vi "Sub01_CommandBuilder.vi"(8 "error in (no error)":errorcluster, 9 "CommandInfo":T1={"RedBall"={"Min"={"G"=0, "B"=0, "R"=160}, "Max"={"G"=160, "B"=160, "R"=255}}, "YellowBall"={"Min"={"G"=140, "B"=0, "R"=140}, "Max"={"G"=255, "B"=175, "R"=255}}, "WhiteBall"={"Min"={"G"=100, "B"=100, "R"=100}, "Max"={"G"=255, "B"=255, "R"=255}}, "BallDiameter"=11, "BackGround"={"Min"={"G"=91, "B"=202, "R"=39}, "Max"={"G"=116, "B"=255, "R"=62}}, "Border"={"Min"={"G"=0, "B"=121, "R"=0}, "Max"={"G"=42, "B"=126, "R"=14}}}, 10 "filenames":string[](array[string]), 11 "path in":path) -> (0 "error out":errorcluster, 3 "String":string)   [LabVIEW 2019]
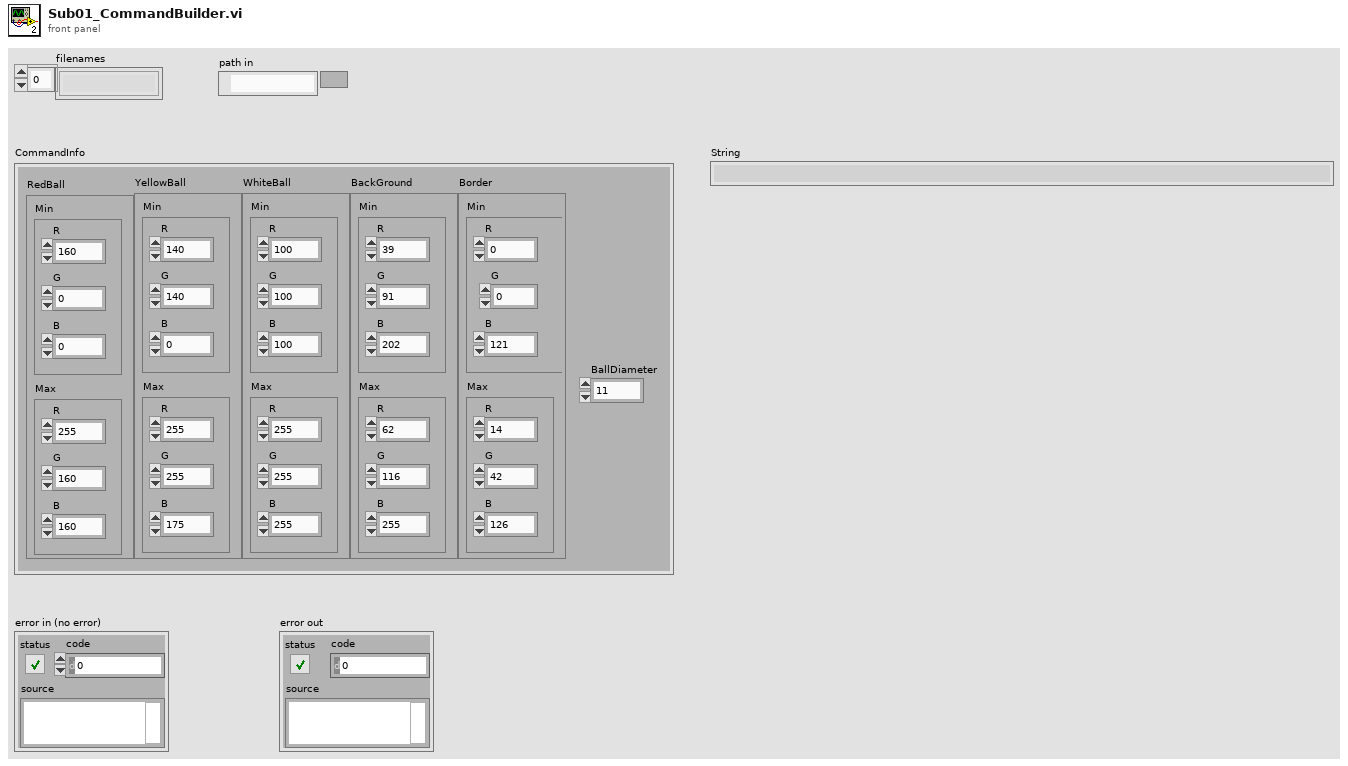
[diagram p1: front panel]
types:
  T1 = cluster{"RedBall":cluster{"Min":cluster{"G":u32, "B":u32, "R":u32}, "Max":cluster{"G":u32, "B":u32, "R":u32}}, "YellowBall":cluster{"Min":cluster{"G":u32, "B":u32, "R":u32}, "Max":cluster{"G":u32, "B":u32, "R":u32}}, "WhiteBall":cluster{"Min":cluster{"G":u32, "B":u32, "R":u32}, "Max":cluster{"G":u32, "B":u32, "R":u32}}, "BallDiameter":u32, "BackGround":cluster{"Min":cluster{"G":u32, "B":u32, "R":u32}, "Max":cluster{"G":u32, "B":u32, "R":u32}}, "Border":cluster{"Min":cluster{"G":u32, "B":u32, "R":u32}, "Max":cluster{"G":u32, "B":u32, "R":u32}}}
  T2 = cluster{"Min":cluster{"G":u32, "B":u32, "R":u32}, "Max":cluster{"G":u32, "B":u32, "R":u32}}
  T3 = typedef "imagedata.ctl" = cluster{"image type":i32, "image depth":i32, "image":u8[], "mask":u8[], "colors":u32[], "Rectangle":cluster{"left":i16, "top":i16, "right":i16, "bottom":i16}}
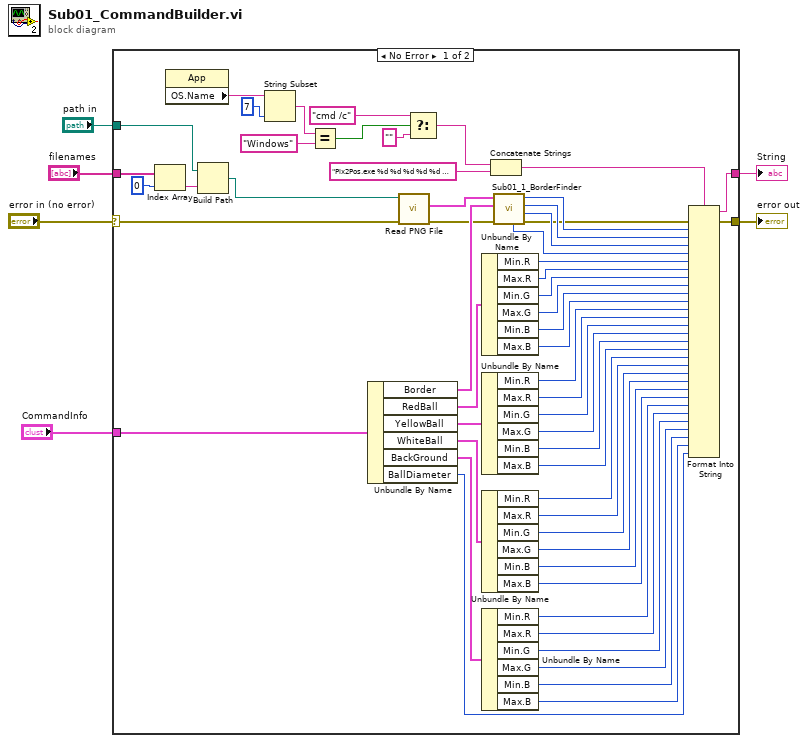
[diagram p0: block diagram]
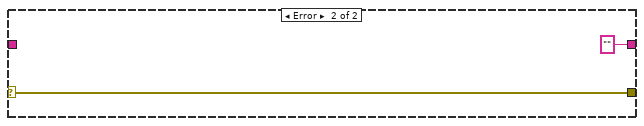
[diagram p2: hidden frame]
diagram:
  n1 = case shown="No Error" "error in (no error)" {
    selector: "error in (no error)" -> [w17 w63]
    tunnel: [w62 w63] -> w6
    tunnel: "filenames" -> [w59 _]
    tunnel: [w58 ""] -> w4
    tunnel: "CommandInfo" -> [w57 _]
    tunnel: "path in" -> [w18 _]
    frame No Error {
      n2 = Index Array(array=w59, index=0) -> (element=w54:string)
      n3 = property class="App"() -> ("OS.Name"=w9:string)  [unwired: 2 in, 2 out]
      n4 = Build Path(base path=w18, name or relative path=w54) -> (appended path=w61:path)
      n5 = String Subset(string=w9, length (rest)=7 ("length (rest)")) -> (substring=w7:string)  [unwired: 1 in]
      n6 = Equal?(x=w7, y="Windows") -> (x = y?=w12:bool)
      n7 = Unbundle By Name(w57) -> ("Border"=w56:T2, "RedBall"=w27:T2, "YellowBall"=w34:T2, "WhiteBall"=w35:T2, "BackGround"=w48:T2, "BallDiameter"=w55:u32)
      n8 = call <vilib>:"Read PNG File.vi"("error in (no error)"=w17, "path to PNG file"=w61) -> ("error out"=w20:errorcluster, "image data"=w53:T3)  [unwired: 7 in, 1 out]
      n9 = Select(t="cmd /c" ("string"), s=w12, f="") -> (s? t:f=w10:string)
      n10 = Unbundle By Name(w27) -> ("Min.R"=w26:u32, "Max.R"=w25:u32, "Min.G"=w24:u32, "Max.G"=w23:u32, "Min.B"=w22:u32, "Max.B"=w21:u32)
      n11 = Unbundle By Name(w34) -> ("Min.R"=w33:u32, "Max.R"=w32:u32, "Min.G"=w31:u32, "Max.G"=w30:u32, "Min.B"=w29:u32, "Max.B"=w28:u32)
      n12 = Unbundle By Name(w35) -> ("Min.R"=w41:u32, "Max.R"=w40:u32, "Min.G"=w39:u32, "Max.G"=w38:u32, "Min.B"=w37:u32, "Max.B"=w36:u32)
      n13 = Unbundle By Name(w48) -> ("Min.R"=w46:u32, "Max.R"=w47:u32, "Min.G"=w45:u32, "Max.G"=w44:u32, "Min.B"=w43:u32, "Max.B"=w42:u32)
      n14 = Concatenate Strings(w10, "Pix2Pos.exe %d %d %d %d %d %d %d %d %d %d %d %d %d %d %d %d %d %d %d %d %d %d %d %d %d %d %d %d %d" ("format string")) -> (w14:string)
      n15 = call "Sub01_1_BorderFinder.vi"("error in (no error)"=w20, "Border"=w56, "image data"=w53) -> ("error out"=w19:errorcluster, "Cmin"=w51:i32, "Lmax"=w50:u32, "Lmin"=w52:i32, "Cmax"=w49:u32)  [unwired: 4 in]
      n16 = Format Into String(format string=w14, error in=w19, w52, w50, w51, w49, w26, w25, w24, w23, w22, w21, w33, w32, w31, w30, w29, w28, w41, w40, w39, w38, w37, w36, w46, w47, w45, w44, w43, w42, w55) -> (resulting string=w58:string, error out=w62:errorcluster)  [unwired: 1 in]
    }
    frame Error {
    }
  }
  "error out" <- w6
  "String" <- w4
